vi "QI_ToggleStreaming.vi"(7 "path to dll":path, 8 "error in (no error)":errorcluster, 10 "Enable?":enum16{"Disable", "Enable"}(ring), 11 "Camera Handle":u32) -> (0 "error out":errorcluster, 1 "enable":u32, 2 "Streaming Error":u32, 3 "Camera Handle":u32)   [LabVIEW 2014]
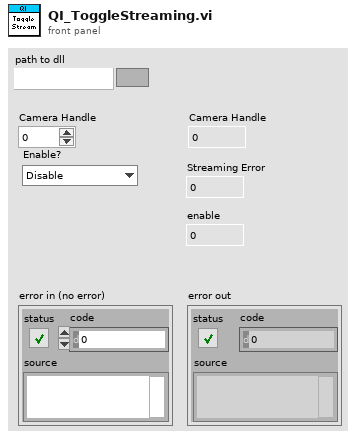
[diagram p1: front panel]
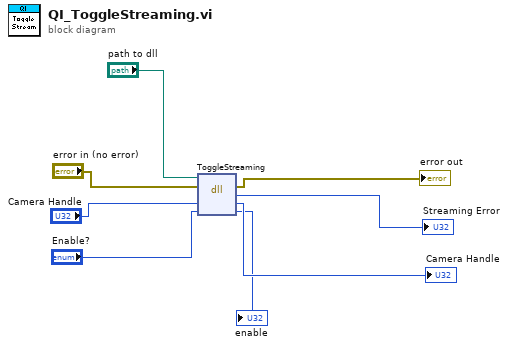
[diagram p0: block diagram]
diagram:
  n1 = dll-call lib="C:/Users/appli/Documents/Aline/octo-labview/QImaging/Release/QImaging.dll" fn="ToggleStreaming"(path in="path to dll", error in="error in (no error)", "handle"="Camera Handle", "enable"="Enable?") -> (error out=→"error out":errorcluster, "return type"=→"Streaming Error":i32, "handle"=→"Camera Handle":u32, "enable"=→"enable":u32)  [unwired: 1 in, 1 out]
